vi "CANPOSITIONBED.vi"() -> ()   [LabVIEW 2009]
uses:
  PWM/PWM_Name.ctl
  FPGA.lvlib
  PWM.lvlib
panel:
  in  "Period (uSec)":u32
  in  "High (uSec)":u32
  in  "PWM":T1=9 items=["Invalid"=0, "PWM1"=1, "PWM2"=2, "PWM9"=9, "PWM10"=10]
  in  "PWM9_Enable":bool
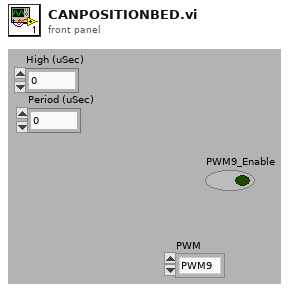
[diagram p1: front panel]
types:
  T1 = typedef "PWM.lvlib/PWM_Name.ctl" = u16
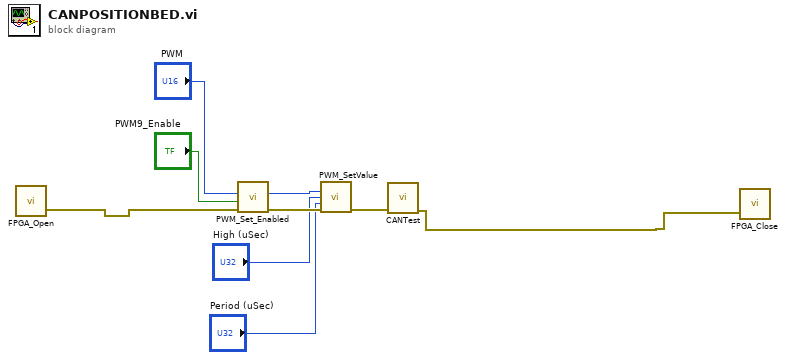
[diagram p0: block diagram]
diagram:
  n1 = call "FPGA_Open.vi"() -> ("error out"=w3:errorcluster)  [unwired: 3 in]
  n2 = call "PWM_Set_Enabled.vi"("error in"=w3, "Enable"="PWM9_Enable", "PWM_in"="PWM") -> ("error out"=w7:errorcluster, "PWM_out"=w6:T1)  [unwired: 7 in]
  n3 = call "PWM_SetValue.vi"("PWM"=w6, "High (uSec)"="High (uSec)", "Period (uSec)"="Period (uSec)", "error in"=w7) -> ("error out"=w2:errorcluster)  [unwired: 11 in]
  n4 = call "CANTest.vi"("error in (no error)"=w2) -> ("error out"=w1:errorcluster)  [unwired: 10 in]
  n5 = call "FPGA_Close.vi"("error in (no error)"=w1) -> ()  [unwired: 2 in, 1 out]
